vi "IZOpen.vi"() -> (1 "PRIORLib.IZOut":refnum<k7>, 2 "error out":errorcluster)   [LabVIEW 2011]
panel:
  in  "PRIORLib.IZ":refnum<k7>
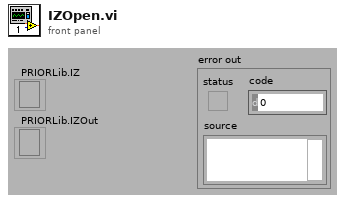
[diagram p1: front panel]
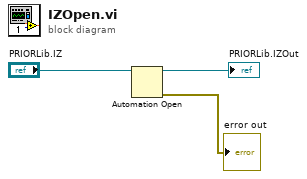
[diagram p0: block diagram]
diagram:
  n1 = Automation Open(Automation Refnum="PRIORLib.IZ") -> (Automation Refnum=→"PRIORLib.IZOut":refnum<k7>, error out=→"error out":errorcluster)  [unwired: 3 in]
